vi "Elapsed_timestamp.vi"(11 "Error in":errorcluster caption="Error in (no error)", 12 "Start time in":timestamp caption="Start time in (0: init)") -> (8 "Elapsed time":dbl caption="Elapsed time [s]" format="%.3f", 13 "Now":timestamp, 14 "Start time out":timestamp, 15 "Error out":errorcluster)   [LabVIEW 2017, in "GPTiming.lvlib"]
doc: "Calculates <B>Elapsed time</B> since <B>Start time in</B>.\n\n<B>Start time in</B> will be returned in <B>Start time out</B>. Set <B>Start time in</B> to a default-valued zero timestamp (or leave it unwired) to get the current time returned in <B>Start time out</B> instead. <B>Now</B> will always be the current time.\n\nThis VI counts time with timestamps and will be able to increase <B>Elapsed time</B> with ms accuracy until the year 3000 (the current maximum year of a LabVIEW timestamp). Using timestamps consume about three times as many CPU-cycles as using the tick counter (it's still measured in nanoseconds), but the timing range is increased tremendously.\n\nThis VI is inlined. <B>Error in</B> is wired straight through to <B>Error out</B> to enable optional dataflow dependency (offering control of when <B>Now</B> is).\n\nSteen Schmidt\nGPower\n5/12 2013"
uses:
  GPTiming.lvlib
panel:
  # "Copyright © 2013\nGPower\nSee enclosed license file for terms and conditions"
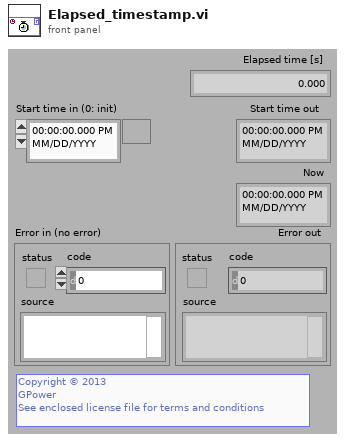
[diagram p1: front panel]
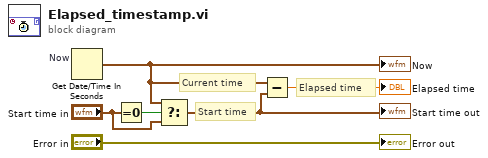
[diagram p0: block diagram]
diagram:
  # "Elapsed time"
  # "Current time"
  # "Start time"
  n1 = Get Date/Time In Seconds "Now"() -> (seconds since 1Jan1904=w1:timestamp)
  "Now" <- w1
  n2 = Equal To 0?(x="Start time in") -> (x = 0?=w6:bool)
  n3 = Select(t=w1, s=w6, f="Start time in") -> (s? t:f=w4:timestamp)
  "Start time out" <- w4
  n4 = Subtract(x=w1, y=w4) -> (x-y=→"Elapsed time":dbl)
  "Error out" <- "Error in"
